vi "saveConfiguration.vi"(8 "error in (no error)":errorcluster, 11 "IDevice in":refnum<class "IDevice.lvclass">) -> (0 "error out":errorcluster, 2 "Configuration out":string, 3 "IDevice out":refnum<class "IDevice.lvclass">)   [LabVIEW 2022 SP3, in "openDAQ.lvlib" / "IBaseObject.lvlib" / "IPropertyObject.lvlib" / "IComponent.lvlib" / "IFolder.lvlib" / "IDevice.lvlib" / "IDevice.lvclass"]
uses:
  <instrlib>/openDAQ/Public/Classes/IDevice/IDevice.lvclass
  <instrlib>/openDAQ/Public/Classes/IDevice/IDevice.lvclass/IDevice.ctl
  <instrlib>/openDAQ/Binaries/Windows/x86/copendaq32.dll
  <instrlib>/openDAQ/Public/Classes/daqCoreTypes/IString/IString.lvclass
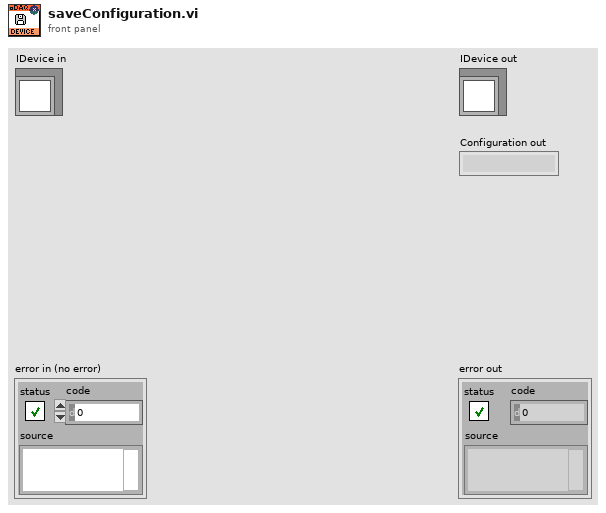
[diagram p1: front panel]
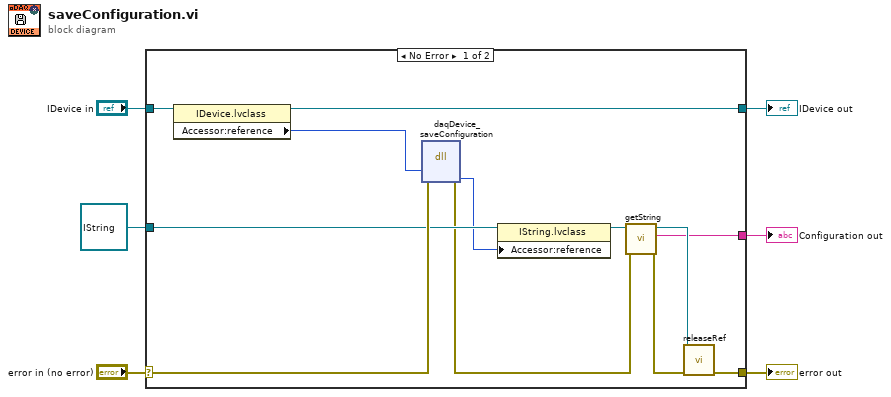
[diagram p0: block diagram]
diagram:
  n1 = case shown="No Error" "error in (no error)" {
    selector: "error in (no error)" -> [w16 w20]
    tunnel: [w9 w20] -> w5
    tunnel: [w15 w19] -> w3
    tunnel: "IDevice in" -> [w18 w19]
    tunnel: refnum<class "IString.lvclass"> refnum ("openDAQ.lvlib:daqCoreTypes.lvlib:IString.lvclass") -> [w14 _]
    tunnel: [w7 _] -> w1
    frame No Error {
      n2 = property class="IDevice.lvclass"(reference=w18) -> (reference out=w15:refnum<class "IDevice.lvclass">, "Accessor:reference"=w17:i64)  [unwired: 1 in, 1 out]
      n3 = dll-call lib="C:/Program Files (x86)/National Instruments/LabVIEW 2022/instr.lib/openDAQ/Binaries/Windows/x86/copendaq*.*" fn="daqDevice_saveConfiguration"(error in=w16, "device"=w17) -> (error out=w11:errorcluster, "arg2"=w13:i64)  [unwired: 5 in, 1 out]
      n4 = property class="IString.lvclass"(reference=w14, "Accessor:reference"=w13) -> (reference out=w12:refnum<class "IString.lvclass">)  [unwired: 1 in, 1 out]
      n5 = call <instrlib>:"getString.vi"("error in (no error)"=w11, "IString in"=w12) -> ("error out"=w10:errorcluster, "String out"=w7:string, "IString out"=w8:refnum<class "IString.lvclass">)  [unwired: 7 in]
      n6 = call-dynamic "releaseRef.vi"("error in (no error)"=w10, "IBaseObject in"=w8) -> ("error out"=w9:errorcluster)  [unwired: 9 in]
    }
    frame Error {
    }
  }
  "error out" <- w5
  "IDevice out" <- w3
  "Configuration out" <- w1
